vi "IP_POWER1_ON_WebSwitch_Control.vi"() -> ()   [LabVIEW 2011]
doc: "Example of using standard HTTP protocol for recieving a web site (the HTML source)\n\n\nThis example uses the GET command. For general information about the HTTP protocol and other commands go to\nhttp://www.w3.org/Protocols\n\n\nBjornar Svingen\nbjornar.svingen@sintef.no bjornar.svingen@ktv.no"
uses:
  Instance           2 37Saved   IP_POWER_ON_WebSwitch_Control .vi
  Instance           6 37Saved   IP_POWER_ON_WebSwitch_Control .vi
panel:
  out "OUT2 CMD 2":string="/state.xml?relay2State=1"
  out "Begin Time":u32
  out "SW OU2 ON/OFF":bool=TRUE
  out "SW OU1 ON/OFF":bool=TRUE
  out "standard output":string
  out "PING WEBSW IP CMD":string
  out "Setup WEBSW IP CMD":string
  out "code":i32
  out "WEBSW_SN":string
  out "WEBSW_IP":string
  out "text":string
  out "Setup Status":bool
  out "result string":string
  out "Device SW State":bool[](array[boolean])
  out "Seach the specific string":string[](array[string])
  out "OUT CMD":string[](array[string])
  out "OUT2 CMD":string="/state.xml?relay2State=1"
  out "OUT1 CMD":string="/state.xml?relay1State=1"
  out "HTML source":string
  # "小心它是110V"
  # "2014-10-8"
  # "Web Switch Control"
  # "需給文檔正確的WebSwitch MAC 與WebSwitch IP"
  # "PowerOn"
  # "POWER1 Relability USE"
  # "Command\nhttp://Device IP/state.xml?relay1State=0\nhttp://Device IP/state.xml?relay1State=1\nhttp://Device IP/state.xml?relay2State=0\nhttp://Device IP/state.xml?relay2State=1"
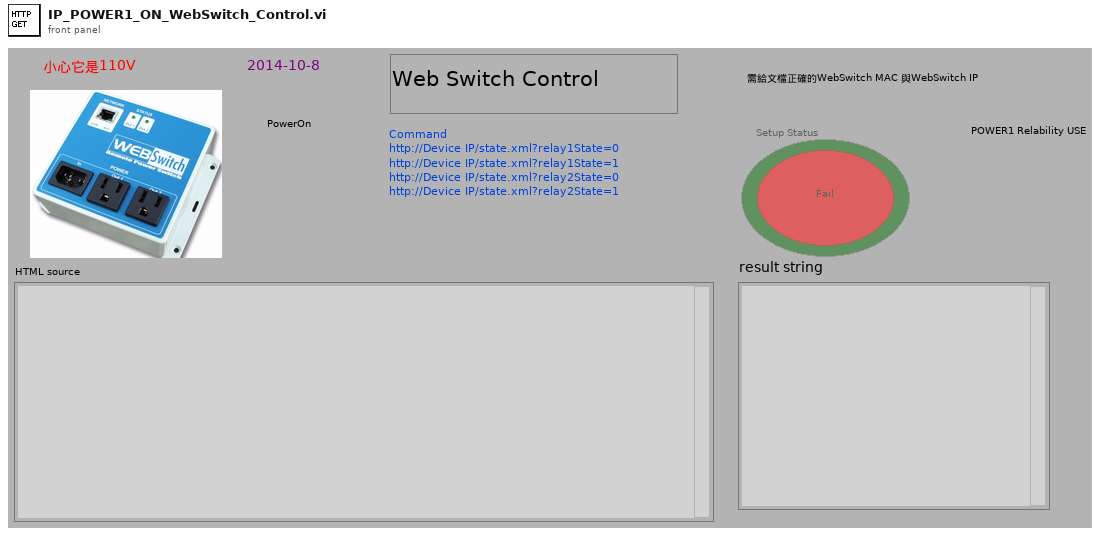
[diagram p1: front panel]
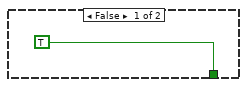
[diagram p5: hidden frame]
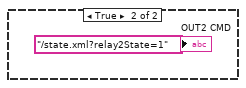
[diagram p7: hidden frame]
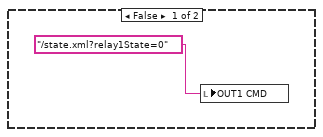
[diagram p8: hidden frame]
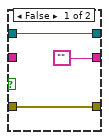
[diagram p9: hidden frame]
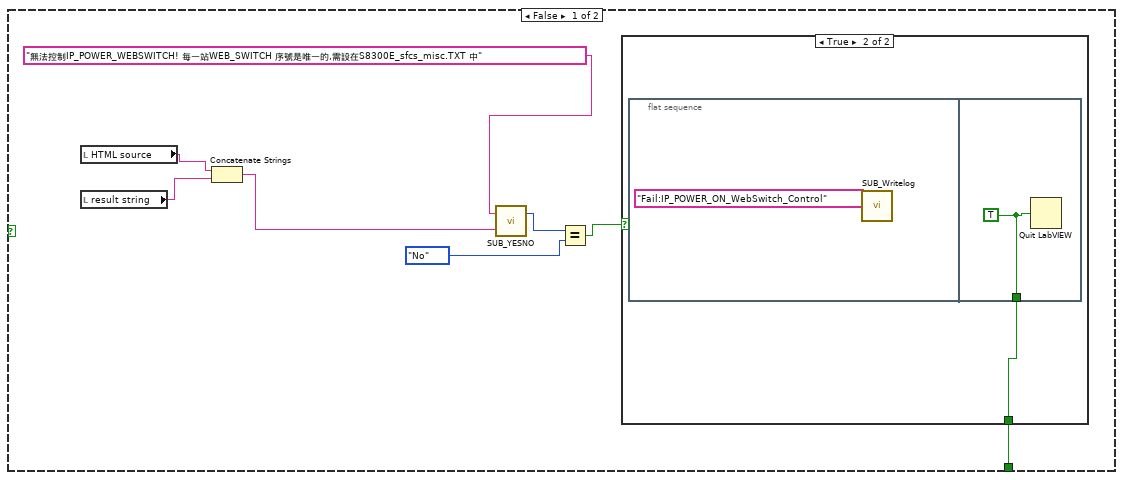
[diagram p10: hidden frame]
diagram:
  n1 = while {
    i -> [w1]
    stop <- w2 stop-if-true
    n2 = flat-sequence {
      tunnel: w1 -> [w4]
      tunnel: [w123] -> w2
      frame #0 {
        n3 = Equal To 0?(x=w4) -> (x = 0?=w3:bool)
        n4 = case shown="True" w3 {
          frame False {
          }
          frame True {
            n5 = Tick Count (ms)() -> (millisecond timer value=→"Begin Time":u32)
          }
        }
      }
      frame #1 {
        w8 = ""
        # "To assign the temporary IP address...\n1. Make sure  WebSwitch TM  and the configuration computer are connected to the same physical\nnetwork.  This will not work through routers or gateways.\n2. Assign the address as follows...\nWindows:\nOpen a Command Prompt (on Windows XP, select START, then RUN, then type “cmd”).\nType...\narp -s {new IP address} {serial number of  WebSwitch TM  }Revision 1.01                           WebSwitch TM    Users Manual\nXytronix Research & Design, Inc.                  page 6\nNote:   IP address format is: xxx.xxx.xxx.xxx\nSerial number format is: ss-ss-ss-ss-ss-ss\nFor example, to set a WebSwitch TM  device (with serial number 00-0C-C8-01-00-01 )  to\n10.10.10.40 the following command would be used.\narp -s 10.10.10.40 00-0c-c8-01-00-01"
        n6 = local write "OUT1 CMD"(w8) -> ()
        n7 = local write "OUT2 CMD"(w8) -> ()
        n8 = local write "result string"(w8) -> ()
        "SW OU1 ON/OFF" <- TRUE ("SW OU1 ON/OFF")
        "SW OU2 ON/OFF" <- FALSE ("SW OU2 ON/OFF")
      }
      frame #2 {
        n9 = call "SUB_SearchFile_inFolder.vi"("Search Filename in Folder"="S8300E_sfcs_misc.TXT") -> ("File Existing True/Flase"=w9:bool)  [unwired: 1 in]
        n10 = case shown="False" w9 {
          frame False {
            n11 = flat-sequence {
              frame #0 {
                n12 = call "Display Message to User2"() -> ()  [unwired: 10 in, 2 out]
              }
              frame #1 {
                n13 = call "SUB_Writelog.vi"("Pass/Fail"="Fail:IP_POWER_ON_WebSwitch_Control") -> ()  [unwired: 2 in]
              }
              frame #2 {
                n14 = Quit LabVIEW(quit? (T)=TRUE) -> ()
              }
            }
          }
          frame True {
          }
        }
      }
      frame #3 {
        n15 = call "SUB_Read_specifFile.vi"("name or relative path"="S8300E_sfcs_misc.TXT") -> ("text"=w19:string)  [unwired: 1 in, 1 out]
        "text" <- w19
        n16 = call "SUB_FindSpecificString.vi"("Find this String"="IP_POWER_WEB_SWITCH_IP=", "String data"=w19) -> ("before \"; \" string"=→"WEBSW_IP":string, "Found"=w17:bool)  [unwired: 2 in]
        n17 = call "SUB_FindSpecificString.vi"("Find this String"="IP_POWER_WEB_SWITCH_SN=", "String data"=w19) -> ("before \"; \" string"=→"WEBSW_SN":string, "Found"=w16:bool)  [unwired: 2 in]
        n18 = And(x=w17, y=w16) -> (x .and. y?=w15:bool)
        n19 = case shown="False" w15 {
          frame False {
            n20 = flat-sequence {
              frame #0 {
                n21 = call "Display Message to User"() -> ()  [unwired: 10 in, 2 out]
              }
              frame #1 {
                n22 = call "SUB_Writelog.vi"("Pass/Fail"="Fail:IP_POWER_ON_WebSwitch_Control") -> ()  [unwired: 2 in]
              }
              frame #2 {
                n23 = Quit LabVIEW(quit? (T)=TRUE) -> ()
              }
            }
          }
          frame True {
          }
        }
      }
      frame #4 {
        n24 = local read "WEBSW_IP"() -> (w26:string)
        n25 = local read "WEBSW_SN"() -> (w29:string)
        n26 = Concatenate Strings("ping -l  102  ", w26, "  -n 1") -> (→"PING WEBSW IP CMD":string)
        n27 = Concatenate Strings("arp -s  ", w26, "  ", w29) -> (→"Setup WEBSW IP CMD":string)
      }
      frame #5 {
        n28 = while {
          stop <- w33 stop-if-true
          n29 = flat-sequence {
            tunnel: [w39] -> w32
            tunnel: [w47] -> w33
            tunnel: w32 -> [w44]
            frame #0 {
              n30 = Concatenate Strings("arp -d *" ("string"), "\r") -> (w35:string)
              n31 = call "SUB_run_exeFile_Textv2.vi"("exe filename"=w35) -> ()  [unwired: 1 in, 2 out]
            }
            frame #1 {
              (unwired) "CMD /C"
              n32 = local read "Setup WEBSW IP CMD"() -> (w40:string)
              n33 = Concatenate Strings(w40, "\r") -> (w38:string)
              n34 = call "SUB_run_exeFile_Textv2.vi"("exe filename"=w38) -> ("code"=w37:i32)  [unwired: 1 in, 1 out]
              "code" <- w37
              n35 = Not Equal To 0?(x=w37) -> (x != 0?=w39:bool)
            }
            frame #2 {
              (unwired) "CMD /C"
              n36 = local read "PING WEBSW IP CMD"() -> (w52:string)
              n37 = Concatenate Strings(w52, "\r") -> (w43:string)
              n38 = call "SUB_run_exeFile_Textv2.vi"("exe filename"=w43) -> ("standard output"=w42:string)  [unwired: 1 in, 1 out]
              "standard output" <- w42
              n39 = call "SUB_FindSpecificString.vi"("Find this String"="Request timed out", "String data"=w42) -> ("Found"=w49:bool)  [unwired: 2 in, 1 out]
              n40 = call "SUB_FindSpecificString.vi"("Find this String"="unreachable", "String data"=w42) -> ("Found"=w48:bool)  [unwired: 2 in, 1 out]
              n41 = Or(x=w49, y=w48) -> (x .or. y?=w46:bool)
              n42 = Or(x=w46, y=w44) -> (x .or. y?=w45:bool)
              n43 = case shown="True" w45 {
                tunnel: [TRUE w55] -> w47
                frame False {
                }
                frame True {
                  n44 = call "SUB_YESNO.vi"("Status"="無法成功Ping WEB Switch ! WEB SW 序號也要設對於文檔S8300E_sfcs_misc.TXT中!") -> ("yes/no"=w57:enum32{"No Selection", "Yes", "No", "None"})  [unwired: 2 in]
                  n45 = Equal?(x=w57, y=enum32{"No Selection", "Yes", "No", "None"}."No") -> (x = y?=w55:bool)
                  n46 = case shown="True" w55 {
                    frame False {
                    }
                    frame True {
                      n47 = flat-sequence {
                        frame #0 {
                          n48 = call "SUB_Writelog.vi"("Pass/Fail"="Fail:IP_POWER_ON_WebSwitch_Control") -> ()  [unwired: 2 in]
                        }
                        frame #1 {
                          n49 = Quit LabVIEW(quit? (T)=TRUE) -> ()
                        }
                      }
                    }
                  }
                }
              }
            }
          }
        }
      }
      frame #6 {
        n50 = local read "SW OU1 ON/OFF"() -> (w62:bool)
        n51 = local read "SW OU2 ON/OFF"() -> (w61:bool)
        n52 = case shown="True" w62 {
          frame False {
            n53 = local write "OUT1 CMD"("/state.xml?relay1State=0") -> ()
          }
          frame True {
            "OUT1 CMD" <- "/state.xml?relay1State=1"
          }
        }
        n54 = case shown="False" w61 {
          frame False {
            n55 = local write "OUT2 CMD"("/state.xml?relay2State=0") -> ()
          }
          frame True {
            "OUT2 CMD" <- "/state.xml?relay2State=1"
          }
        }
      }
      frame #7 {
        (unwired) FALSE
        (unwired) "relay2state1"
        n56 = local read "OUT2 CMD"() -> (→"OUT2 CMD 2":string)
        n57 = local read "OUT1 CMD"() -> (w73:string)
        n58 = Build Array(FALSE) -> (→"Device SW State":bool[])
        n59 = Build Array("relay1state1") -> (→"Seach the specific string":string[])
        n60 = Build Array(w73) -> (→"OUT CMD":string[])
      }
      frame #8 {
      }
      frame #9 {
        n61 = for {
          N: 1 -> [_]
          i -> [w85]
          # "Compose the header\n(can include lots of things, see www.w3.org/Protodols)"
          # "The GET method is used to recieve a website.\n\nThe header is composed according to the HTTP 1.1 standard"
          # "Close the connection"
          # "If error code=66, meaning the server\nhas transferred all the data and closed\nthe connection, treat this error as no error."
          # "Read the reply\n(from the GET method)\nin 1024 byte blocks\nand stop on any error."
          # "Write the \"header\"\nto the web site"
          # "Open TCP connection at\nspecifyed web site"
          n62 = local read "WEBSW_IP"() -> (w75:string)
          n63 = TCP Open Connection(address=w75, remote port or service name=u16 80 ("remote port")) -> (connection ID=w81:refnum<k5>, error out=w80:errorcluster)  [unwired: 3 in]
          n64 = local read "OUT CMD"() -> (w92:string[])
          n65 = call <vilib>:"Trim Whitespace.vi"("string"=w75) -> ("trimmed string"=w95:string)  [unwired: 1 in]
          n66 = Index Array(array=w92, index=w85) -> (element=w91:string)
          n67 = call <vilib>:"Trim Whitespace.vi"("string"=w91) -> ("trimmed string"=w99:string)  [unwired: 1 in]
          n68 = local read "Seach the specific string"() -> (w90:string[])
          n69 = Concatenate Strings("GET " ("Command"), w99, " HTTP/1.1" ("Command"), "\r\n" ("string"), "Host: " ("Command"), w95, "\r\n\r\n" ("string")) -> (w93:string)
          n70 = TCP Write(connection ID=w81, data in=w93, error in (no error)=w80) -> (connection ID out=w107:refnum<k5>, error out=w106:errorcluster)  [unwired: 1 in, 1 out]
          n71 = while {
            tunnel: w106 -> [w121]
            tunnel: w107 -> [w120]
            tunnel: [w116] -> w104
            tunnel: [w119] -> w101
            tunnel: [w118] -> w103 mode=indexing
            stop <- w116 stop-if-true
            n72 = TCP Read(connection ID=w120, bytes to read=1024, error in (no error)=w121) -> (connection ID out=w119:refnum<k5>, data out=w118:string, error out=w116:errorcluster)  [unwired: 2 in]
          }
          n73 = Index Array(array=w90, index=w85) -> (element=w87:string)
          n74 = Unbundle By Name(w104) -> ("code"=w109:i32)
          n75 = Concatenate Strings(w103) -> (w102:string)
          n76 = Equal?(x=w109, y=66) -> (x = y?=w108:bool)
          n77 = local read "Device SW State"() -> (w86:bool[])
          n78 = case shown="True" w108 {
            tunnel: ["" w114] -> w89
            tunnel: w102 -> [_ w114]
            tunnel: [w111 errorcluster {"status"=FALSE, "code"=0, "source"=""} ("error in (no error)")] -> w76
            tunnel: w104 -> [w111 _]
            tunnel: w101 -> [w110 w113]
            tunnel: [w110 w113] -> w78
            frame False {
            }
            frame True {
            }
          }
          "HTML source" <- w89
          n79 = TCP Close Connection(connection ID=w78, abort (F)=TRUE, error in (no error)=w76) -> (error out=w79:errorcluster)  [unwired: 1 out]
          n80 = call <vilib>:"Simple Error Handler.vi"("error in (no error)"=w79) -> ()  [unwired: 4 in, 5 out]
          n81 = call "SUB_OUT_String_token.vi"("input string"=w89) -> ("result string"=w88:string)  [unwired: 2 in]
          "result string" <- w88
          n82 = call "SUB_FindSpecificString.vi"("Find this String"=w87, "String data"=w88) -> ("Found"=w84:bool)  [unwired: 2 in, 1 out]
          n83 = Replace Array Subset(array=w86, new element=w84, index=w85) -> (w83:bool[])
          n84 = local write "Device SW State"(w83) -> ()
        }
      }
      frame #10 {
      }
      frame #11 {
        n85 = local read "Device SW State"() -> (w130:bool[])
        n86 = local read "SW OU1 ON/OFF"() -> (w126:bool)
        n87 = Index Array(array=w130) -> (element #1=w129:bool, element #2=w128:bool)  [unwired: 2 in]
        n88 = local read "SW OU2 ON/OFF"() -> (w125:bool)
        n89 = Equal?(x=w126, y=w129) -> (x = y?=w127:bool)
        n90 = Equal?(x=w125, y=w128) -> ()  [unwired: 1 out]
        n91 = And(x=w127, y=TRUE) -> (x .and. y?=w124:bool)
        "Setup Status" <- w124
        n92 = case shown="True" w124 {
          tunnel: [w131 w142] -> w123
          frame False {
            n93 = local read "HTML source"() -> (w137:string)
            n94 = local read "result string"() -> (w136:string)
            n95 = Concatenate Strings(w137, w136) -> (w135:string)
            n96 = call "SUB_YESNO.vi"("Debug View"=w135, "Status"="無法控制IP_POWER_WEBSWITCH! 每一站WEB_SWITCH 序號是唯一的,需設在S8300E_sfcs_misc.TXT 中") -> ("yes/no"=w134:enum32{"No Selection", "Yes", "No", "None"})  [unwired: 1 in]
            n97 = Equal?(x=w134, y=enum32{"No Selection", "Yes", "No", "None"}."No") -> (x = y?=w132:bool)
            n98 = case shown="True" w132 {
              tunnel: [_ w139] -> w131
              frame False {
              }
              frame True {
                n99 = flat-sequence {
                  tunnel: [w141] -> w139
                  frame #0 {
                    n100 = call "SUB_Writelog.vi"("Pass/Fail"="Fail:IP_POWER_ON_WebSwitch_Control") -> ()  [unwired: 2 in]
                  }
                  frame #1 {
                    w141 = TRUE ("quit? (T)")
                    n101 = Quit LabVIEW(quit? (T)=w141) -> ()
                  }
                }
              }
            }
          }
          frame True {
            n102 = flat-sequence {
              tunnel: [w149] -> w142
              frame #0 {
                n103 = local read "Begin Time"() -> (w148:u32)
                n104 = Tick Count (ms)() -> (millisecond timer value=w144:u32)
                n105 = call "SUB_CAL_TESTTIME.vi"("Test Item name"="IP_POWER_ON_WebSwitch_Control", "Stop tick time"=w144, "Start tick time"=w148) -> ("Test Time output"=w146:string)  [unwired: 2 in]
                n106 = Concatenate Strings("Pass:IP_POWER_ON_WebSwitch_Control", w146) -> (w145:string)
                n107 = call "SUB_Writelog.vi"("Pass/Fail"=w145) -> ()  [unwired: 2 in]
              }
              frame #1 {
                w149 = TRUE ("quit? (T)")
                n108 = Quit LabVIEW(quit? (T)=w149) -> ()
              }
            }
          }
        }
      }
    }
  }
